vi "getValueFromXMLNative.vi"(8 "error in (no error)":errorcluster, 10 "eventXML":refnum<k20>, 11 "ScriptEvent in":refnum<class "ScriptEvent.lvclass">) -> (0 "error out":errorcluster, 2 "eventXML out":refnum<k20>, 3 "ScriptEvent out":refnum<class "ScriptEvent.lvclass">)   [LabVIEW 2009, in "Tools.lvlib" / "Scripting.lvlib" / "ScriptEvent.lvclass"]
uses:
  ScriptEvent.lvclass
  <vilib>/xml/Close Reference(Node).vi
  ScriptEvent.lvclass/ScriptEvent.ctl
  <vilib>/xml/NI_XML.lvlib
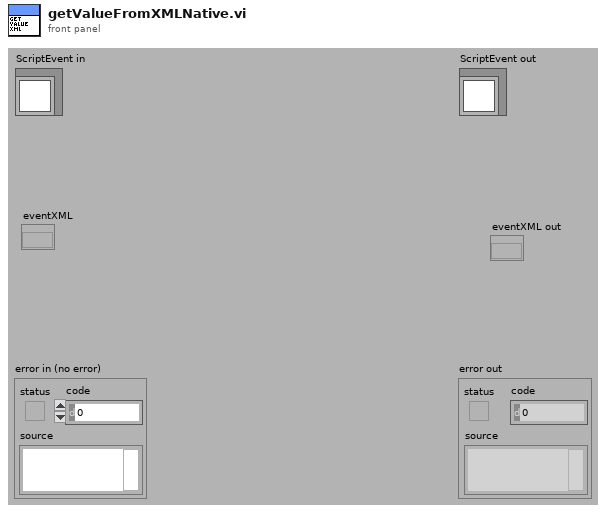
[diagram p1: front panel]
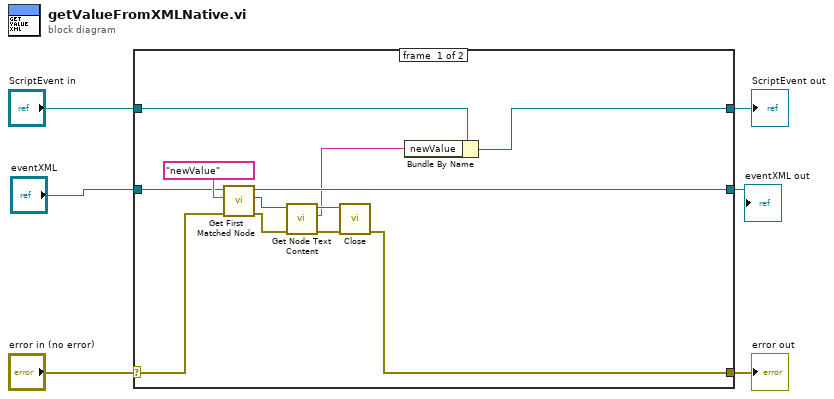
[diagram p0: block diagram]
diagram:
  n1 = case shown="No Error" "error in (no error)" {
    selector: "error in (no error)" -> [w11 w20]
    tunnel: [w7 w20] -> w5
    tunnel: [w8 w19] -> w3
    tunnel: "ScriptEvent in" -> [w9 w19]
    tunnel: "eventXML" -> [w13 _]
    tunnel: [w12 _] -> w1
    frame #0 {
      n2 = call <vilib>:"Get First Matched Node.vi"("error in (no error)"=w11, "XPath expression"="newValue", "node in"=w13) -> ("error out"=w17:errorcluster, "node result"=w16:refnum<k20>, "node out"=w12:refnum<k20>)  [unwired: 6 in]
      n3 = call <vilib>:"Get Node Text Content.vi"("error in (no error)"=w17, "node in"=w16) -> ("error out"=w15:errorcluster, "node text"=w10:string, "node out"=w14:refnum<k20>)  [unwired: 7 in]
      n4 = call-poly <vilib>:"Close.vi"("error in (no error)"=w15, "node"=w14) -> ("error out"=w7:errorcluster)  [unwired: 7 in]
      n5 = Bundle By Name(cluster=w9, "newValue"=w10) -> (w8:refnum<class "ScriptEvent.lvclass">)
    }
    frame #1 {
    }
  }
  "error out" <- w5
  "ScriptEvent out" <- w3
  "eventXML out" <- w1
